vi "OpenFrontPanel.vi"(8 "ErrorIn":errorcluster, 11 "ObjectIn":refnum<class "FrontPanelControl.lvclass">) -> (0 "ErrorOut":errorcluster, 3 "ObjectOut":refnum<class "FrontPanelControl.lvclass">)   [LabVIEW 2021, in "FrontPanelControl.lvclass"]
uses:
  FrontPanelControl.lvclass
  FrontPanelControl.lvclass/FrontPanelControl.ctl
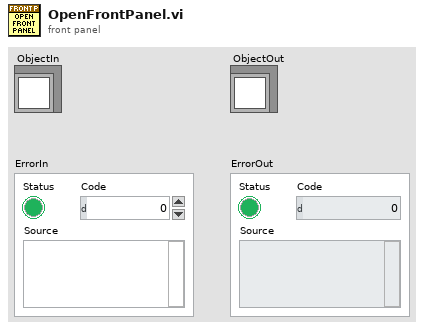
[diagram p1: front panel]
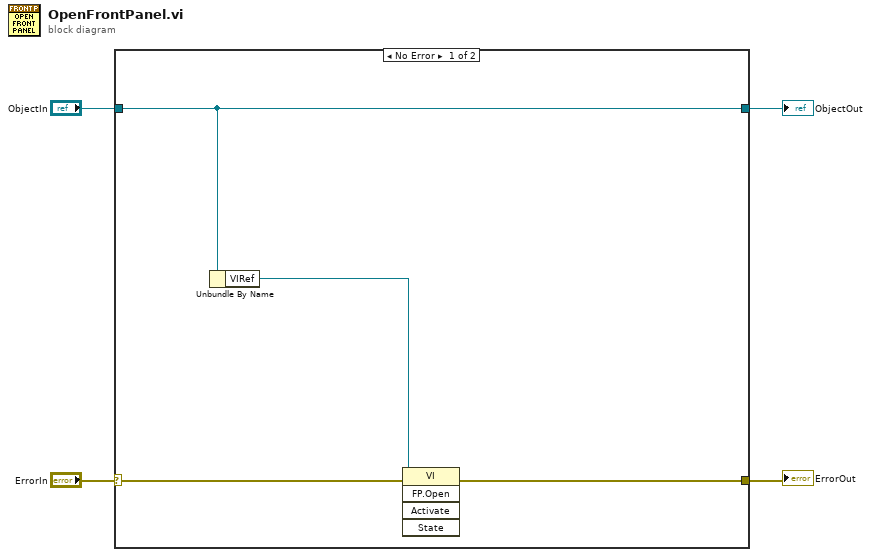
[diagram p0: block diagram]
diagram:
  n1 = case shown="No Error" "ErrorIn" {
    selector: "ErrorIn" -> [w8 w10]
    tunnel: [w7 w10] -> w3
    tunnel: [w6 w9] -> w1
    tunnel: "ObjectIn" -> [w6 w9]
    frame No Error {
      n2 = Unbundle By Name(w6) -> ("VIRef"=w5:refnum<vi>)
      n3 = invoke class="VI" method="FP.Open"(reference=w5, error in=w8) -> (error out=w7:errorcluster)  [unwired: 3 in, 4 out]
    }
    frame Error {
    }
  }
  "ErrorOut" <- w3
  "ObjectOut" <- w1
